vi "Event buffer.vi"() -> ()   [LabVIEW 2021]
uses:
  <vilib>/DAQmx/write.llb/DAQmx Write (Analog DBL 1Chan 1Samp).vi
  <vilib>/DAQmx/read.llb/DAQmx Read (Analog 1D DBL 1Chan NSamp).vi
  <vilib>/DAQmx/create/channels.llb/DAQmx Create Channel (AI-Voltage-Basic).vi
  <vilib>/DAQmx/configure/timing.llb/DAQmx Timing (Sample Clock).vi
  <vilib>/DAQmx/create/channels.llb/DAQmx Create Channel (AO-Voltage-Basic).vi
  <vilib>/DAQmx/miscellaneous.llb/DAQmx Fill In Error Info.vi
panel:
  out "sampleInterval":u32
  out "timed out":bool
  out "Loop Writer":i32
  out "Loop reader":i32
  in  "Slide":dbl(slide) scale=-5.0..5.0
  in  "stop 2":bool
  out "Waveform Chart":dbl[](graph)
  in  "stop":bool
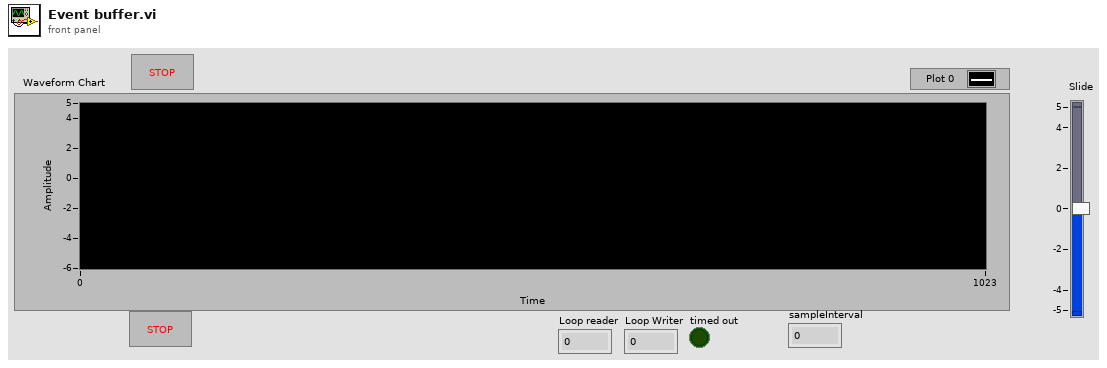
[diagram p1: front panel]
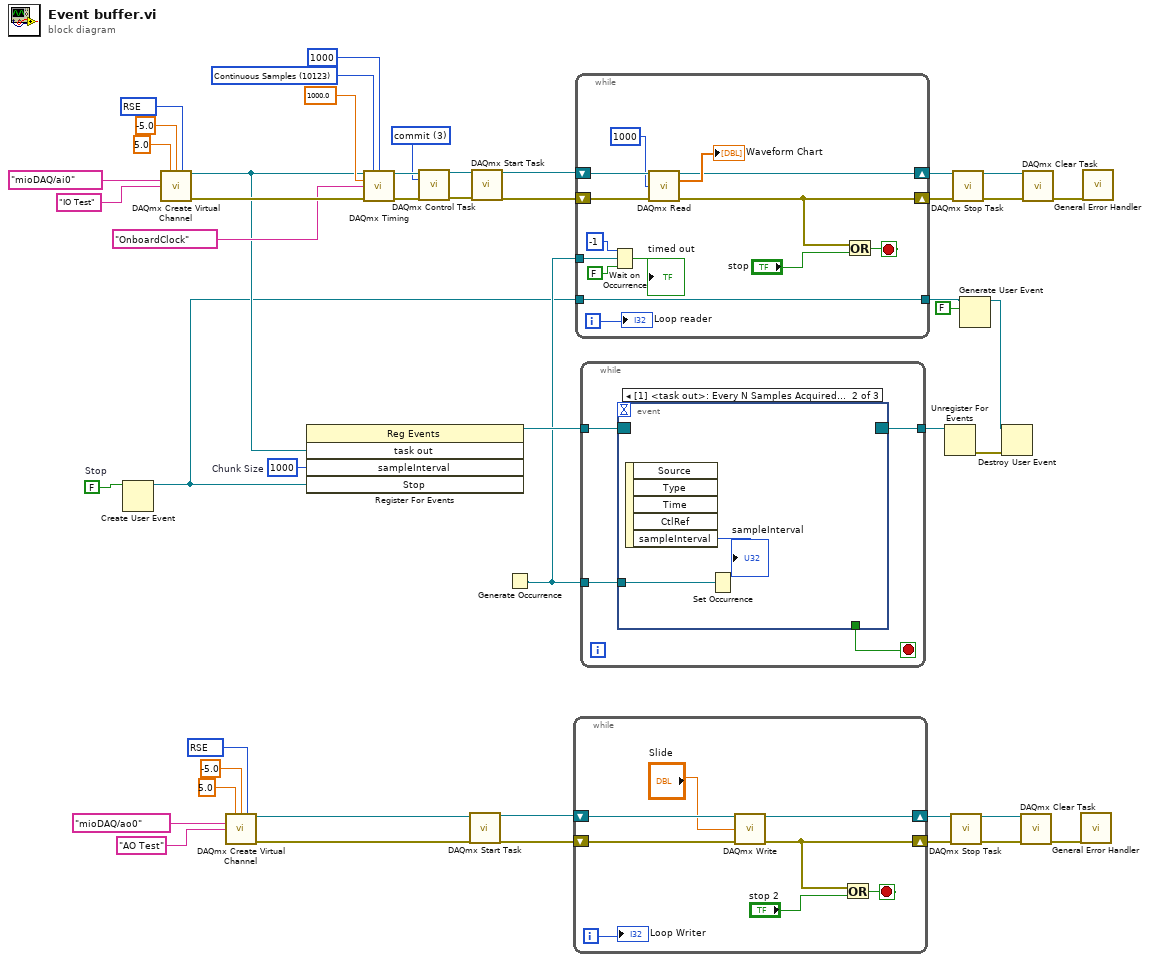
[diagram p0: block diagram]
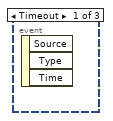
[diagram p2: hidden frame]
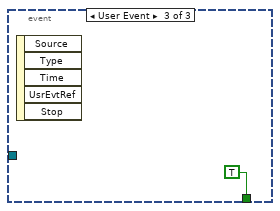
[diagram p3: hidden frame]
diagram:
  w6 = FALSE  # Stop
  w8 = u32 1000  # Chunk Size
  w12 = 10083 items=["Default"=-1, "RSE"=10083, "Differential"=10106, "Pseudodifferential"=12529] ("output terminal configuration")
  w13 = 10083 items=["Default"=-1, "RSE"=10083, "NRSE"=10078, "Differential"=10106, "Pseudodifferential"=12529] ("input terminal configuration")
  w29 = 3 items=["verify"=2, "reserve"=4, "commit"=3, "unreserve"=5, "abort"=6] ("action")
  w41 = 10123 items=["Finite Samples"=10178, "Continuous Samples"=10123, "Hardware Timed Single Point"=12522] ("sample mode")
  n1 = Create User Event(user event datatype=w6) -> (user event=w5:refnum<user-event>)  [unwired: 1 in, 1 out]
  n2 = call-poly <vilib>:"DAQmx Create Virtual Channel.vi"("maximum value"=5.0, "minimum value"=-5.0, "input terminal configuration"=w13, "physical channels"=tag "mioDAQ/ai0", "name to assign"="IO Test") -> ("task out"=w9:refnum<k21>, "error out"=w47:errorcluster)  [unwired: 9 in]
  n3 = call-poly <vilib>:"DAQmx Create Virtual Channel.vi"("maximum value"=5.0, "minimum value"=-5.0, "output terminal configuration"=w12, "physical channels"=tag "mioDAQ/ao0", "name to assign"="AO Test") -> ("task out"=w15:refnum<k21>, "error out"=w16:errorcluster)  [unwired: 9 in]
  n4 = register-events(w9, w8, w5) -> (reference out=w10:refnum<event-registration>)  [unwired: 2 in, 1 out]
  n5 = call-poly <vilib>:"DAQmx Timing.vi"("task/channels in"=w9, "sample mode"=w41, "samples per channel"=1000, "rate"=1000.0, "source"=tag "OnboardClock", "error in"=w47) -> ("task out"=w33:refnum<k21>, "error out"=w32:errorcluster)  [unwired: 8 in]
  n6 = call <vilib>:"DAQmx Control Task.vi"("task/channels in"=w33, "action"=w29, "error in"=w32) -> ("task out"=w31:refnum<k21>, "error out"=w30:errorcluster)  [unwired: 11 in]
  n7 = call <vilib>:"DAQmx Start Task.vi"("task/channels in"=w15, "error in"=w16) -> ("task out"=w25:refnum<k21>, "error out"=w26:errorcluster)  [unwired: 12 in]
  n8 = call <vilib>:"DAQmx Start Task.vi"("task/channels in"=w31, "error in"=w30) -> ("task out"=w28:refnum<k21>, "error out"=w27:errorcluster)  [unwired: 12 in]
  n9 = Generate Occurrence() -> (w7:refnum<k4>)
  n10 = while {
    shift-right: [w53] -> w17
    shift-left: w25 -> [w55]
    shift-right: [w51] -> w18
    shift-left: w26 -> [w54]
    i -> [w48]
    stop <- w50 stop-if-true
    n11 = call-poly <vilib>:"DAQmx Write.vi"("task/channels in"=w55, "data"="Slide", "error in"=w54) -> ("task out"=w53:refnum<k21>, "error out"=w51:errorcluster)  [unwired: 10 in, 1 out]
    n12 = Or(x=w51, y="stop 2") -> (x .or. y?=w50:bool)
    "Loop Writer" <- w48
  }
  n13 = while {
    shift-right: [w63] -> w46
    shift-left: w28 -> [w69]
    shift-right: [w66] -> w45
    shift-left: w27 -> [w68]
    tunnel: w7 -> [w61]
    tunnel: w5 -> [w59]
    tunnel: [w59] -> w4
    i -> [w62]
    stop <- w65 stop-if-true
    n14 = Wait on Occurrence(1:FALSE ("ignore previous (T)"), 2:w61, 3:-1 ("ms timeout (-1)")) -> (0:→"timed out":bool)
    n15 = call-poly <vilib>:"DAQmx Read.vi"("task/channels in"=w69, "number of samples per channel"=1000, "error in"=w68) -> ("task out"=w63:refnum<k21>, "data"=→"Waveform Chart":dbl[], "error out"=w66:errorcluster)  [unwired: 10 in]
    n16 = Or(x=w66, y="stop") -> (x .or. y?=w65:bool)
    "Loop reader" <- w62
  }
  n17 = while {
    tunnel: [w73] -> w11
    tunnel: w10 -> [w72]
    tunnel: w7 -> [w71]
    stop <- w70 stop-if-true
    n18 = event shown="[1] <task out>: Every N Samples Acquired into Buffer" {
      selector: w72 -> [_ _ _]
      dyn-events: [_ _ _] -> w73
      timeout: _ -> [_ _ _]
      tunnel: w71 -> [_ w75 _]
      tunnel: [_ _ TRUE] -> w70
      event Timeout {
        n19 = event-data() -> ()  [unwired: 1 in, 3 out]
      }
      event Every N Samples Acquired into Buffer {
        n20 = event-data() -> ("sampleInterval"=→"sampleInterval":u32)  [unwired: 1 in, 4 out]
        n21 = Set Occurrence(w75) -> ()
      }
      event User Event {
        n22 = event-data() -> ()  [unwired: 1 in, 5 out]
      }
    }
  }
  n23 = Unregister For Events(event registration refnum=w11) -> (error out=w3:errorcluster)  [unwired: 1 in]
  n24 = call <vilib>:"DAQmx Stop Task.vi"("task/channels in"=w17, "error in"=w18) -> ("task out"=w19:refnum<k21>, "error out"=w20:errorcluster)  [unwired: 12 in]
  n25 = call <vilib>:"DAQmx Stop Task.vi"("task/channels in"=w46, "error in"=w45) -> ("task out"=w44:refnum<k21>, "error out"=w43:errorcluster)  [unwired: 12 in]
  n26 = Generate User Event(user event=w4, event data cluster=FALSE ("event data")) -> (user event out=w2:refnum<user-event>)  [unwired: 2 in, 1 out]
  n27 = Destroy User Event(user event=w2, error in=w3) -> ()  [unwired: 1 out]
  n28 = call <vilib>:"DAQmx Clear Task.vi"("task in"=w19, "error in"=w20) -> ("error out"=w21:errorcluster)  [unwired: 13 in]
  n29 = call <vilib>:"DAQmx Clear Task.vi"("task in"=w44, "error in"=w43) -> ("error out"=w42:errorcluster)  [unwired: 13 in]
  n30 = call <vilib>:"General Error Handler.vi"("error in (no error)"=w21) -> ()  [unwired: 10 in, 5 out]
  n31 = call <vilib>:"General Error Handler.vi"("error in (no error)"=w42) -> ()  [unwired: 10 in, 5 out]
